vi "Debug_FilterColumn.vi"(11 "Array in":string[](array[string])) -> (3 "Array out":string[](array[string]))   [LabVIEW 2017, in "Server.lvlib" / "Message Queue.lvlib"]
doc: "This VI gets a whole Column containing Strings and deletes Duplicates. Its used to display e.g. all Queues that occured in a List for a User Menu"
uses:
  Message Queue.lvlib
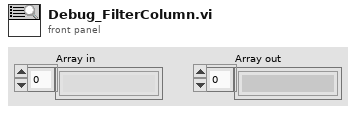
[diagram p1: front panel]
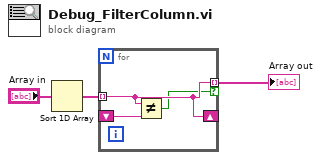
[diagram p0: block diagram]
diagram:
  n1 = Sort 1D Array(array="Array in") -> (sorted array=w2:string[])
  n2 = for {
    tunnel: w2 -> [w5] mode=indexing
    shift-right: [w5] -> _
    shift-left: _ -> [w6]
    tunnel: [w5] -> w3 mode=indexing if=w4
    n3 = Not Equal?(x=w5, y=w6) -> (x != y?=w4:bool)
  }
  "Array out" <- w3
